vi "SendTriggerPulse.vi"(10 "Trigger Duration (ms)":u32=25, 11 "Refnum in":refnum<k21>) -> (3 "Refnum out":refnum<k21>)   [LabVIEW 2013]
uses:
  <vilib>/DAQmx/write.llb/DAQmx Write (Digital Bool 1Line 1Point).vi
  <vilib>/DAQmx/miscellaneous.llb/DAQmx Fill In Error Info.vi
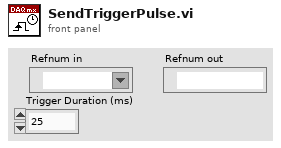
[diagram p1: front panel]
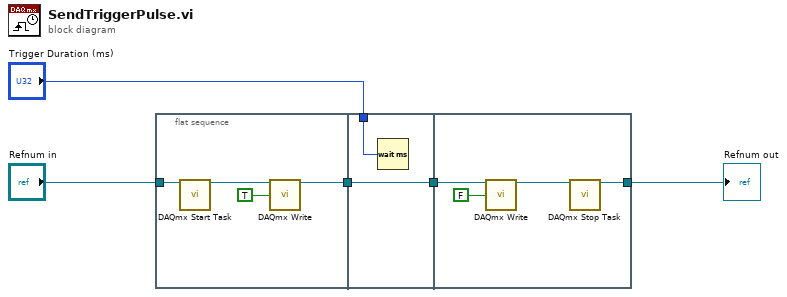
[diagram p0: block diagram]
diagram:
  n1 = flat-sequence {
    tunnel: [w8] -> w3
    tunnel: "Refnum in" -> [w6]
    tunnel: w3 -> [w11]
    tunnel: [w11] -> w2
    tunnel: "Trigger Duration (ms)" -> [w10]
    tunnel: w2 -> [w15]
    tunnel: [w12] -> w5
    frame #0 {
      n2 = call <vilib>:"DAQmx Start Task.vi"("task/channels in"=w6) -> ("task out"=w7:refnum<k21>)  [unwired: 13 in, 1 out]
      n3 = call-poly <vilib>:"DAQmx Write.vi"("task/channels in"=w7, "data"=TRUE) -> ("task out"=w8:refnum<k21>)  [unwired: 11 in, 2 out]
    }
    frame #1 {
      n4 = Wait (ms)(milliseconds to wait=w10) -> ()  [unwired: 1 out]
    }
    frame #2 {
      n5 = call-poly <vilib>:"DAQmx Write.vi"("task/channels in"=w15, "data"=FALSE) -> ("task out"=w13:refnum<k21>)  [unwired: 11 in, 2 out]
      n6 = call <vilib>:"DAQmx Stop Task.vi"("task/channels in"=w13) -> ("task out"=w12:refnum<k21>)  [unwired: 13 in, 1 out]
    }
  }
  "Refnum out" <- w5
